vi "EcrireLireValeurParDefaut.vi"(7 "Lecture/Ecriture":enum32{"Lecture", "Ecriture"}(radio), 8 "error in (no error)":errorcluster, 11 "defParametersIN":T1={"customParam"={"CamDelayToOpen(µs)"=10, "FLWidth(µs)"=10, "QSWidth(µs)"=10, "DelayFL_QS (µs)"=180, "CamDelayToClose(µs)"=100, "CamPivExposure(µs)"=100}, "Configuration"={"Nombre de période"=2, "Fréquence "=0, "Nb pulse préchauffe laser"=41248, "skip_frame_PIV"=0, "skip_frame_LAT"=0, "Time beetwen pulses (µs)"=2, "Temps LAT (µs)"=0, "Temps expo LAT (µs)"=100000, "action"=enum."PIV + LAT"}}) -> (0 "error out":errorcluster, 2 "XML File Path(duplicate)":path, 3 "defParametersOUT":T1={"customParam"={"CamDelayToOpen(µs)"=10, "FLWidth(µs)"=10, "QSWidth(µs)"=10, "DelayFL_QS (µs)"=180, "CamDelayToClose(µs)"=100, "CamPivExposure(µs)"=100}, "Configuration"={"Nombre de période"=2, "Fréquence "=0, "Nb pulse préchauffe laser"=41248, "skip_frame_PIV"=0, "skip_frame_LAT"=0, "Time beetwen pulses (µs)"=2, "Temps LAT (µs)"=0, "Temps expo LAT (µs)"=100000, "action"=enum."PIV + LAT"}})   [LabVIEW 2023]
uses:
  defaultParam.ctl
  customParam.ctl
  configUtilisateur.ctl
  <vilib>/Utility/xml.llb/Read From XML File(string).vi
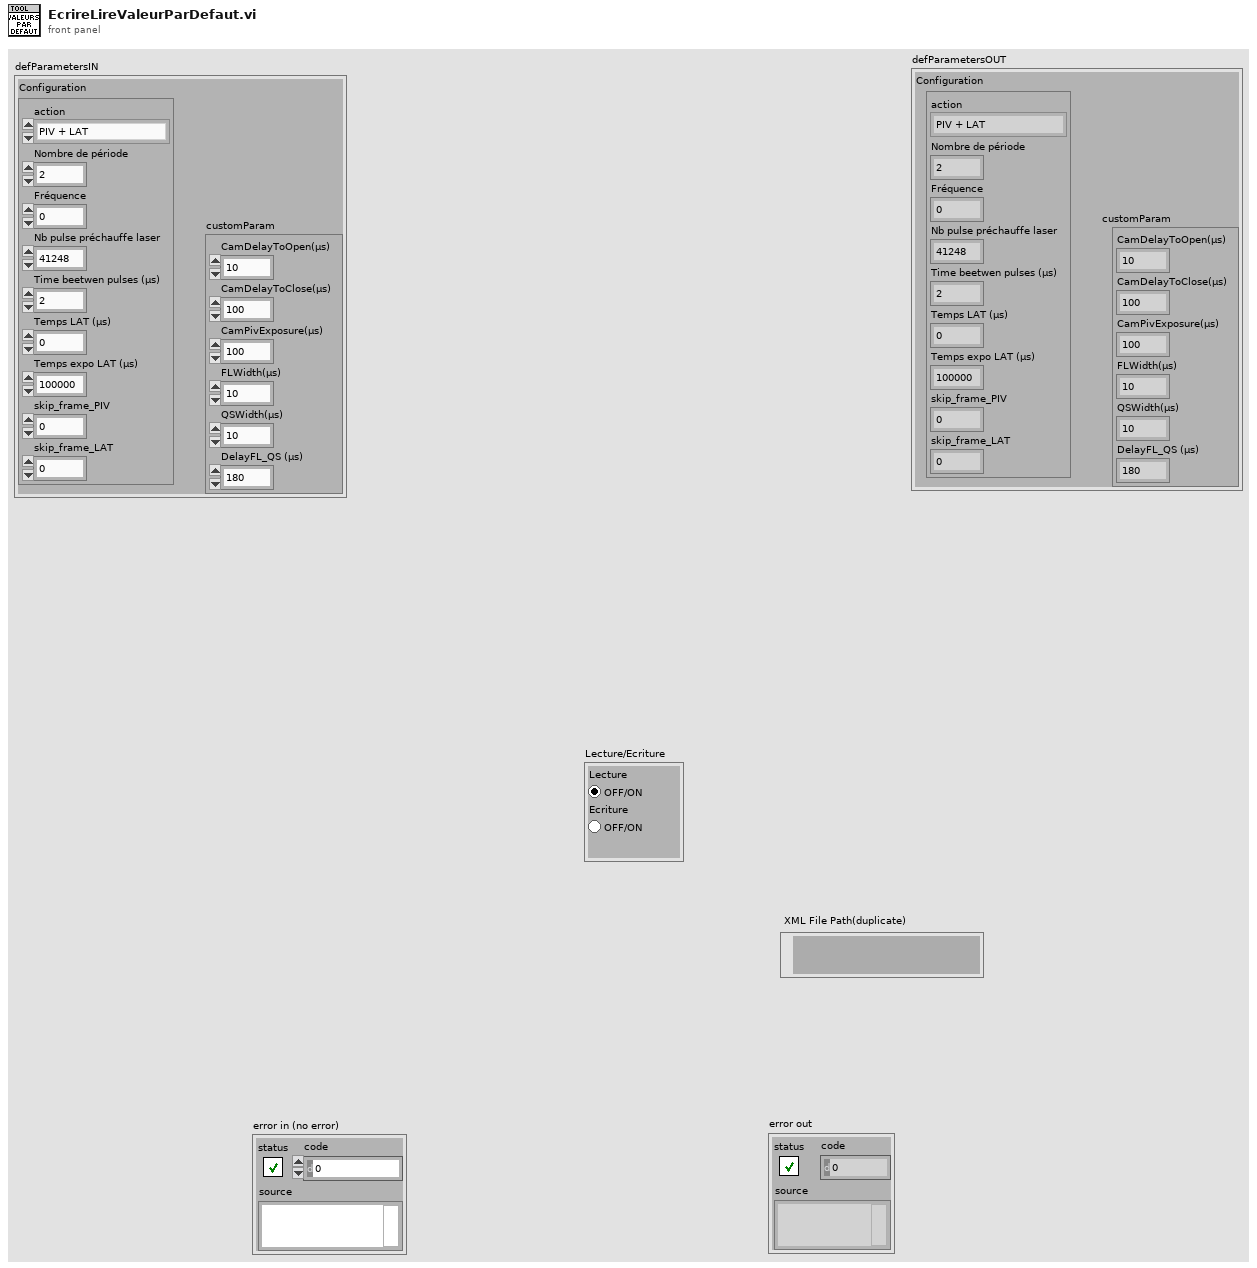
[diagram p1: front panel]
types:
  T1 = typedef "defaultParam.ctl" = cluster{"customParam":T2, "Configuration":T3}
  T2 = typedef "customParam.ctl" = cluster{"CamDelayToOpen(µs)":u32, "FLWidth(µs)":u32, "QSWidth(µs)":u32, "DelayFL_QS (µs)":u32, "CamDelayToClose(µs)":u32, "CamPivExposure(µs)":u32}
  T3 = typedef "configUtilisateur.ctl" = cluster{"Nombre de période":u16, "Fréquence ":u16, "Nb pulse préchauffe laser":u16, "skip_frame_PIV":u8, "skip_frame_LAT":u8, "Time beetwen pulses (µs)":u32, "Temps LAT (µs)":u32, "Temps expo LAT (µs)":u32, "action":enum8{"PIV", "PIV + LAT", "LAT"}}
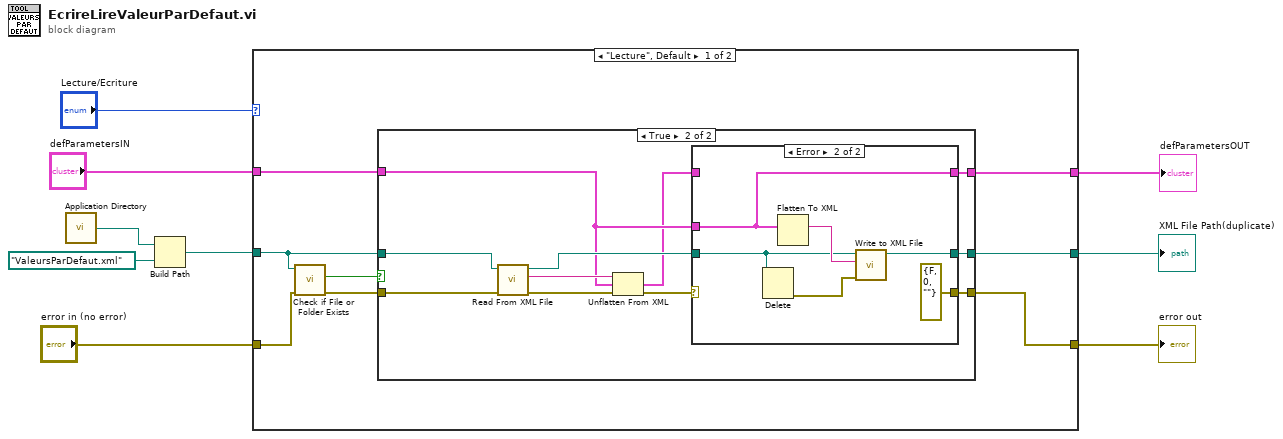
[diagram p0: block diagram]
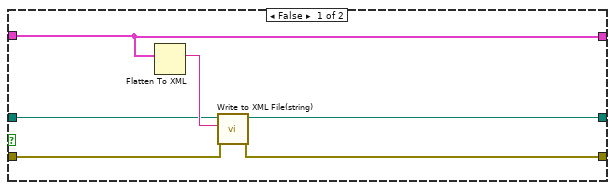
[diagram p2: hidden frame]
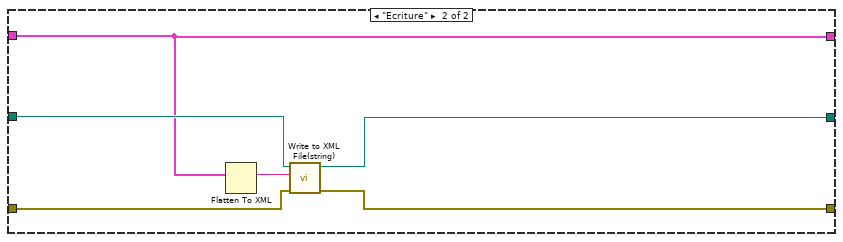
[diagram p4: hidden frame]
diagram:
  n1 = call <vilib>:"Application Directory.vi"() -> ("Application Directory"=w3:path)
  n2 = Build Path(base path=w3, name or relative path=path "ValeursParDefaut.xml" ("default name")) -> (appended path=w8:path)
  n3 = case shown="\"Lecture\", Default" "Lecture/Ecriture" {
    tunnel: w8 -> [w15 w48]
    tunnel: "error in (no error)" -> [w14 w47]
    tunnel: [w16 w46] -> w6
    tunnel: [w17 w45] -> w5
    tunnel: "defParametersIN" -> [w11 w44]
    tunnel: [w10 w44] -> w1
    frame "Lecture", Default {
      n4 = call <vilib>:"Check if File or Folder Exists.vi"("error in (no error)"=w14, "path"=w15) -> ("error out"=w13:errorcluster, "file or folder exists?"=w12:bool)  [unwired: 7 in, 1 out]
      n5 = case shown="True" w12 {
        tunnel: [w18 w25] -> w10
        tunnel: [w19 w29] -> w17
        tunnel: [w21 w27] -> w16
        tunnel: w15 -> [w20 w32]
        tunnel: w13 -> [w22 w31]
        tunnel: w11 -> [w18 w26]
        frame False {
          n6 = Flatten To XML(6:w18) -> (2:w23:string)
          n7 = call-poly <vilib>:"Write to XML File(string).vi"("error in (no error)"=w22, "XML Input"=w23, "XML File Path"=w20) -> ("error out"=w21:errorcluster, "XML File Path(duplicate)"=w19:path)  [unwired: 2 in, 5 out]
        }
        frame True {
          n8 = call-poly <vilib>:"Read From XML File.vi"("error in (no error)"=w31, "XML File Path"=w32) -> ("error out"=w34:errorcluster, "XML Elements"=w33:string, "XML File Path(duplicate)"=w28:path)  [unwired: 7 in]
          n9 = Unflatten From XML(xml string=w33, type=w26, error in (no error)=w34) -> (value=w24:T1, error out=w30:errorcluster)
          n10 = case shown="Error" w30 {
            selector: w30 -> [w36 _]
            tunnel: [w37 w42] -> w29
            tunnel: w28 -> [w37 w39]
            tunnel: [w36 errorcluster {"status"=FALSE, "code"=0, "source"=""} ("error IO")] -> w27
            tunnel: w26 -> [_ w40]
            tunnel: [w35 w40] -> w25
            tunnel: w24 -> [w35 _]
            frame No Error {
            }
            frame Error {
              n11 = Delete(path (use dialog)=w39) -> (error out=w38:errorcluster)  [unwired: 4 in, 2 out]
              n12 = Flatten To XML(6:w40) -> (2:w41:string)
              n13 = call-poly <vilib>:"Write to XML File.vi"("error in (no error)"=w38, "XML Input"=w41, "XML File Path"=w39) -> ("XML File Path(duplicate)"=w42:path)  [unwired: 2 in, 6 out]
            }
          }
        }
      }
    }
    frame "Ecriture" {
      n14 = Flatten To XML(6:w44) -> (2:w49:string)
      n15 = call-poly <vilib>:"Write to XML File(string).vi"("error in (no error)"=w47, "XML Input"=w49, "XML File Path"=w48) -> ("error out"=w46:errorcluster, "XML File Path(duplicate)"=w45:path)  [unwired: 2 in, 5 out]
    }
  }
  "error out" <- w6
  "XML File Path(duplicate)" <- w5
  "defParametersOUT" <- w1
